vi "DrawMultipleLines.vi"(0 "reference in":refnum<class "LcPictureBox.lvclass">, 1 "LineEndPoints":cluster{"x":sgl, "y":sgl}[](array[cluster]), 3 "Color(Black)":u32(colorbox), 4 "Alpha(100%)":dbl=100.0 min=0.0 max=100.0 format="%#_g%%", 5 "Error In":errorcluster, 7 "Fill(False)":bool, 8 "SmoothingMode(AntiAlias)":T1=enum."AntiAlias", 9 "Pen(Width=1, Solid)":T2={"Width"=1, "Style"=enum."Solid"}) -> (14 "reference out":refnum<class "LcPictureBox.lvclass">, 19 "Error Out":errorcluster)   [LabVIEW 2020, in "LcPictureBox.lvclass"]
uses:
  LcPictureBox.lvclass
  System.Drawing
  Pen.ctl
  SmoothingMode.ctl
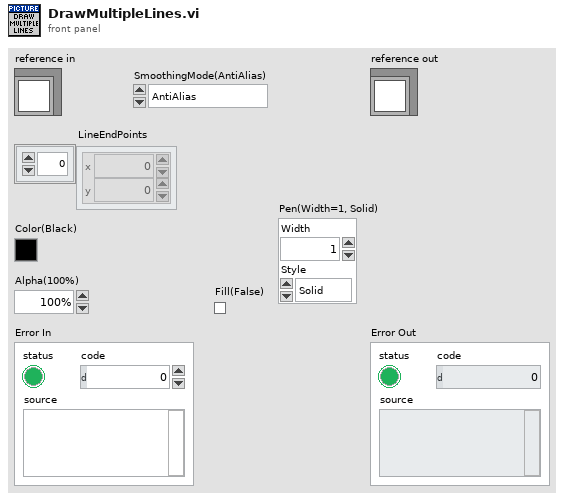
[diagram p1: front panel]
types:
  T1 = typedef "LcPictureBox.lvclass/SmoothingMode.ctl" = enum16{"None", "HighSpeed", "HighQuality", "AntiAlias"}
  T2 = typedef "LcPictureBox.lvclass/Pen.ctl" = cluster{"Width":u16, "Style":enum32{"Solid", "Dash", "Dot", "DashDot", "DashDotDot"}}
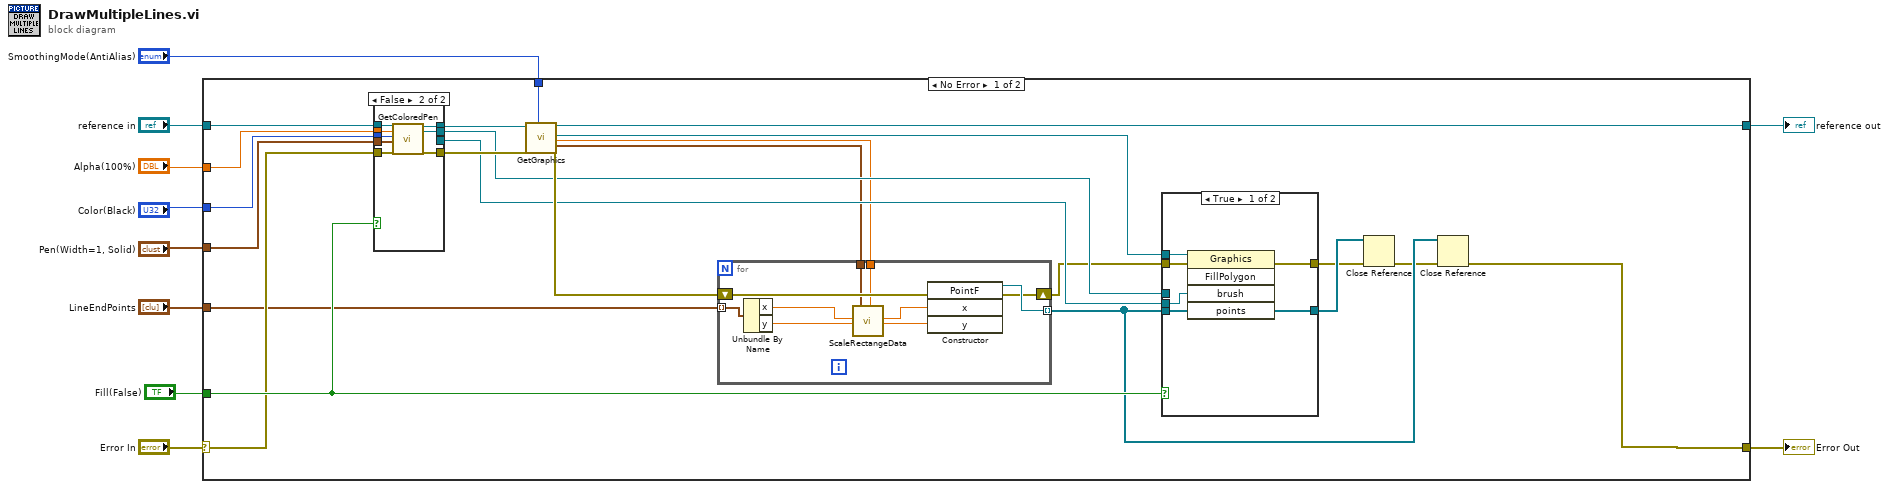
[diagram p0: block diagram]
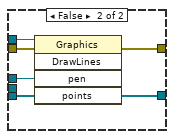
[diagram p2: hidden frame]
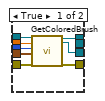
[diagram p3: hidden frame]
diagram:
  n1 = case shown="No Error" "Error In" {
    selector: "Error In" -> [w25 w73]
    tunnel: [w21 w73] -> w9
    tunnel: [w32 w72] -> w7
    tunnel: "reference in" -> [w19 w72]
    tunnel: "SmoothingMode(AntiAlias)" -> [w30 _]
    tunnel: "Color(Black)" -> [w28 _]
    tunnel: "Alpha(100%)" -> [w29 _]
    tunnel: "Pen(Width=1, Solid)" -> [w27 _]
    tunnel: "LineEndPoints" -> [w20 _]
    tunnel: "Fill(False)" -> [w26 _]
    frame No Error {
      n2 = case shown="False" w26 {
        tunnel: [w63 w71] -> w24
        tunnel: w19 -> [w62 w70]
        tunnel: w25 -> [w61 w69]
        tunnel: [w60 w68] -> w23
        tunnel: w29 -> [w59 w67]
        tunnel: w28 -> [w58 w66]
        tunnel: w27 -> [w57 w65]
        tunnel: [_ w64] -> w18
        tunnel: [w56 _] -> w22
        frame True {
          n3 = call "GetColoredBrush.vi"("reference in"=w62, "Alpha(100%)"=w59, "Color(Black)"=w58, "Pen(Width=1, Solid)"=w57, "Error In"=w61) -> ("reference out"=w63:refnum<class "LcPictureBox.lvclass">, "SolidBrushRef"=w56:refnum<k24>, "Error Out"=w60:errorcluster)  [unwired: 12 in]
        }
        frame False {
          n4 = call "GetColoredPen.vi"("reference in"=w70, "Alpha(100%)"=w67, "Color(Black)"=w66, "Pen(Width=1, Solid)"=w65, "Error In"=w69) -> ("reference out"=w71:refnum<class "LcPictureBox.lvclass">, "PenRef"=w64:refnum<k24>, "Error Out"=w68:errorcluster)  [unwired: 12 in]
        }
      }
      n5 = call "GetGraphics.vi"("LcPictureBox in"=w24, "error in (no error)"=w23, "SmoothingMode"=w30) -> ("LcPictureBox out"=w32:refnum<class "LcPictureBox.lvclass">, "Graphics"=w31:refnum<k24>, "Scale"=w12:sgl, "Offset"=w11:cluster{"x":sgl, "y":sgl}, "error out"=w33:errorcluster)  [unwired: 12 in]
      n6 = for {
        tunnel: w20 -> [w55] mode=indexing
        tunnel: [w54] -> w16 mode=indexing
        shift-right: [w52] -> w17
        shift-left: w33 -> [w53]
        tunnel: w12 -> [w47]
        tunnel: w11 -> [w46]
        n7 = Unbundle By Name(w55) -> ("x"=w51:sgl, "y"=w50:sgl)
        n8 = call "ScaleRectangeData.vi"("X-In"=w51, "Y-In"=w50, "Offset(raw)"=w46, "Scale"=w47) -> ("X-Out"=w48:sgl, "Y-Out"=w49:sgl)  [unwired: 12 in, 2 out]
        n9 = constructor class="PointF"(error in=w53, "x"=w48, "y"=w49) -> (reference out=w54:refnum<k24>, error out=w52:errorcluster)  [unwired: 2 in, 3 out]
      }
      n10 = case shown="True" w26 {
        tunnel: w17 -> [w39 w45]
        tunnel: [w38 w44] -> w13
        tunnel: w16 -> [w37 w43]
        tunnel: w18 -> [_ w42]
        tunnel: w31 -> [w36 w41]
        tunnel: w22 -> [w35 _]
        tunnel: [w34 w40] -> w15
        frame True {
          n11 = invoke class="Graphics" method="FillPolygon"(reference=w36, error in=w39, "brush"=w35, "points"=w37) -> (error out=w38:errorcluster, "points"=w34:refnum<k24>[])  [unwired: 1 in, 3 out]
        }
        frame False {
          n12 = invoke class="Graphics" method="DrawLines"(reference=w41, error in=w45, "pen"=w42, "points"=w43) -> (error out=w44:errorcluster, "points"=w40:refnum<k24>[])  [unwired: 1 in, 3 out]
        }
      }
      n13 = Close Reference(reference=w15, error in (no error)=w13) -> (error out=w14:errorcluster)
      n14 = Close Reference(reference=w16, error in (no error)=w14) -> (error out=w21:errorcluster)
    }
    frame Error {
    }
  }
  "Error Out" <- w9
  "reference out" <- w7
